vi "hts_queue.vi"() -> (0 "error out":errorcluster, 3 "Queue out":refnum<queue>)   [LabVIEW 2013]
uses:
  main_machine/type_defs/hts_message.ctl
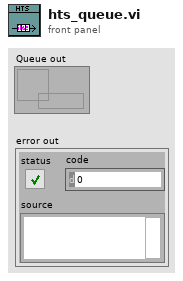
[diagram p1: front panel]
types:
  T1 = typedef "hts_message.ctl" = enum16{"INITIALIZE", "REMOVE CULTURE", "DILUTE AND INDUCE", "SAMPLE REACTOR", "CLEAR LINES", "MOVE TO NEXT", "SHUTDOWN"}
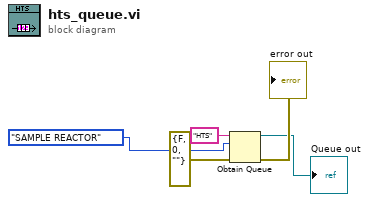
[diagram p0: block diagram]
diagram:
  n1 = Obtain Queue(name (unnamed)="HTS", element data type=hts_message."SAMPLE REACTOR" ("COMMAND"), error in (no error)=errorcluster {"status"=FALSE, "code"=0, "source"=""}) -> (queue out=→"Queue out":refnum<queue>, error out=→"error out":errorcluster)  [unwired: 2 in, 1 out]
